vi "Input DMA Engine.vi"(8 "error in (no error)":errorcluster, 10 "Parameters":T1={"Waveform Ref"=refnum, "DMA Ref"=refnum, "Write to VS Engine.Refs"={"Refs"=[], "Values"=[]}, "Write to VS Engine.FIFO"=refnum, "Name"="", "DMA Settings"={"Number of Channels"=0, "Delacing Scheme"=enum."Interlaced", "Update Rate"=0, "dt"=1000.0}} {"DMA Settings"."dt" format="%#_p"; "DMA Settings"."Update Rate" items=["1 Hz"=1, "2 Hz"=2, "5 Hz"=5, "10 Hz"=10]; "Write to VS Engine.Refs"."Refs" format="%.0x"}, 11 "Parent":string) -> (0 "error out":errorcluster)   [LabVIEW 2015, in "FPGA Addon Engine.lvlib"]
uses:
  FPGA Addon Engine.lvlib
  Types/DMA Input References.ctl
  <vilib>/NI VeriStand/Custom Device Waveform API/Multiple Waveforms Write (DBL)/Multiple Waveforms Write (DBL).lvclass
  Types/DMA Input Ref.ctl
  <vilib>/NI Veristand/Custom Device API/Data Reference.ctl
  Shared/DMA Settings.ctl
  Shared/Delacing Scheme.ctl
  <vilib>/NI Veristand/Custom Device Waveform API/Multiple Waveforms Write (DBL)/NI VeriStand - Close Multiple Waveforms Write Session (DBL).vi
  <vilib>/FPGAPlugInAG/Dynamic/niLvFpga_Close_Dynamic.vi
  <vilib>/rvi/interface/nirviCloseFPGA/nirviCloseFPGA.xnode
  <vilib>/NI VeriStand/Custom Device Waveform API/NI_VS Custom Device Waveform API.lvlib
  Error Handling API/Error Handling API.lvlib
  <vilib>/NI Veristand/Custom Device Tools/Custom Device Utility Library/Custom Device Utility Library.lvlib
  Inline Async API/Inline Async API.lvlib
  <vilib>/NI VeriStand/Custom Device API/Custom Device API.lvlib
  Shared/FPGA Addon Shared.lvlib
panel:
  in  "stop":bool
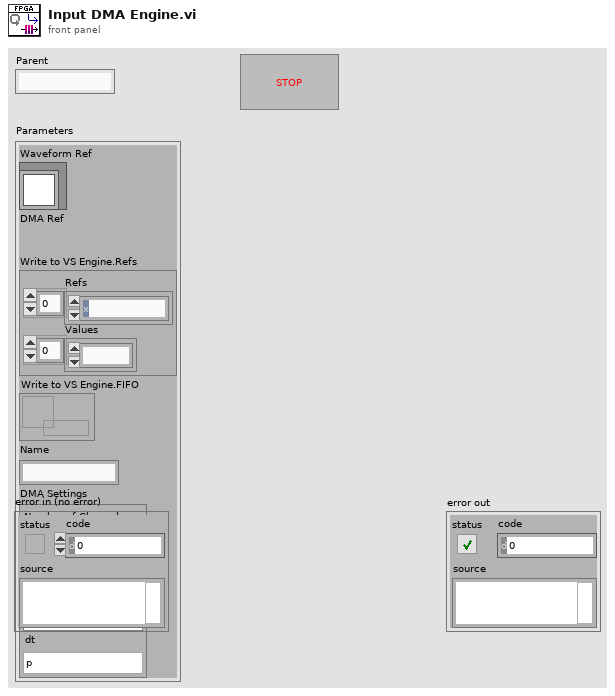
[diagram p1: front panel]
types:
  T1 = typedef "FPGA Addon Engine.lvlib/DMA Input References.ctl" = cluster{"Waveform Ref":refnum<class "Multiple Waveforms Write (DBL).lvclass">, "DMA Ref":T2, "Write to VS Engine.Refs":cluster{"Refs":T3[], "Values":dbl[]}, "Write to VS Engine.FIFO":refnum<k33>, "Name":string, "DMA Settings":T4}
  T2 = typedef "FPGA Addon Engine.lvlib/DMA Input Ref.ctl" = refnum<k20>
  T3 = typedef "Custom Device API.lvlib/Data Reference.ctl" = i32
  T4 = typedef "FPGA Addon Shared.lvlib/DMA Settings.ctl" = cluster{"Number of Channels":u8, "Delacing Scheme":T5, "Update Rate":u32, "dt":dbl}
  T5 = typedef "FPGA Addon Shared.lvlib/Delacing Scheme.ctl" = enum8{"Interlaced"}
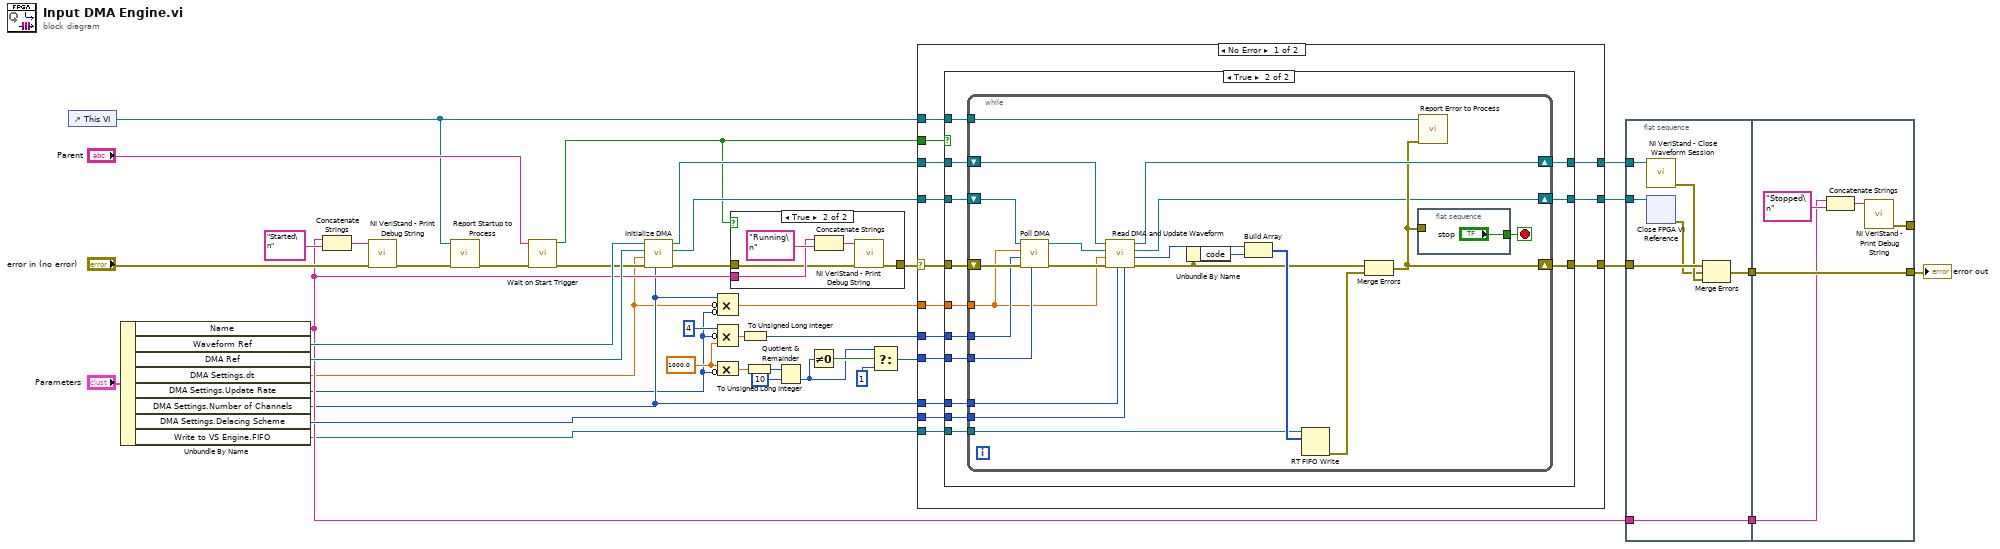
[diagram p0: block diagram]
diagram:
  w6 = 1000.0 ("y")
  n1 = control-ref of="This VI"() -> (w32:refnum<vi>)
  n2 = Unbundle By Name("Parameters") -> ("Name"=w10:string, "Waveform Ref"=w39:refnum<class "Multiple Waveforms Write (DBL).lvclass">, "DMA Ref"=w18:T2, "DMA Settings.dt"=w3:dbl, "DMA Settings.Update Rate"=w2:u32, "DMA Settings.Number of Channels"=w4:u8, "DMA Settings.Delacing Scheme"=w19:T5, "Write to VS Engine.FIFO"=w9:refnum<k33>)
  n3 = Concatenate Strings(w10, "Started\n" ("string")) -> (w29:string)
  n4 = call <vilib>:"NI VeriStand - Print Debug String.vi"("error in (no error)"="error in (no error)", "Message"=w29) -> ("error out"=w17:errorcluster)  [unwired: 9 in]
  n5 = call "Report Startup to Process.vi"("Error"=w17, "This VI"=w32) -> ("error out"=w31:errorcluster)  [unwired: 9 in]
  n6 = call "Wait on Start Trigger.vi"("error in (no error)"=w31, "Name"="Parent") -> ("error out"=w14:errorcluster, "notification"=w15:bool)  [unwired: 8 in]
  n7 = call "Initialize DMA.vi"("Number of Channels"=w4, "error in (no error)"=w14, "dt"=w3, "DMA Ref"=w18, "Multiple Waveforms Write (DBL) in"=w39) -> ("error out"=w13:errorcluster, "DMA Ref"=w37:T2, "Multiple Waveforms Write (DBL) out"=w38:refnum<class "Multiple Waveforms Write (DBL).lvclass">)  [unwired: 4 in]
  n8 = Compound Arithmetic op=MULTIPLY(w4, invert w3, invert w2) -> (w1:dbl)
  n9 = Compound Arithmetic op=MULTIPLY(u32 4 ("value"), invert w2, w6) -> (w7:dbl)
  n10 = Compound Arithmetic op=MULTIPLY(w6, invert w2) -> (w21:dbl)
  n11 = case shown="True" w15 {
    tunnel: w10 -> [_ w44]
    tunnel: w13 -> [w41 w43]
    tunnel: [w41 w42] -> w12
    frame False {
    }
    frame True {
      n12 = Concatenate Strings(w44, "Running\n" ("string")) -> (w46:string)
      n13 = call <vilib>:"NI VeriStand - Print Debug String.vi"("error in (no error)"=w43, "Message"=w46) -> ("error out"=w42:errorcluster)  [unwired: 9 in]
    }
  }
  n14 = To Unsigned Long Integer(number=w7) -> (unsigned 32bit integer=w5:u32)
  n15 = To Unsigned Long Integer(number=w21) -> (unsigned 32bit integer=w24:u32)
  n16 = Quotient & Remainder(x=w24, y=u32 10) -> (floor(x/y)=w20:u32)  [unwired: 1 out]
  n17 = Not Equal To 0?(x=w20) -> (x != 0?=w27:bool)
  n18 = Select(t=w20, s=w27, f=u32 1) -> (s? t:f=w8:u32)
  n19 = case shown="No Error" w12 {
    selector: w12 -> [w52 w101]
    tunnel: w38 -> [w60 w100]
    tunnel: w37 -> [w59 w99]
    tunnel: w1 -> [w58 _]
    tunnel: w4 -> [w57 _]
    tunnel: [w56 w100] -> w36
    tunnel: [w55 w101] -> w35
    tunnel: w5 -> [w54 _]
    tunnel: w32 -> [w53 _]
    tunnel: w15 -> [w51 _]
    tunnel: w8 -> [w50 _]
    tunnel: [w49 w99] -> w23
    tunnel: w19 -> [w48 _]
    tunnel: w9 -> [w47 _]
    frame No Error {
      n20 = case shown="True" w51 {
        tunnel: w60 -> [w63 w76]
        tunnel: w59 -> [w61 w75]
        tunnel: w58 -> [_ w74]
        tunnel: w57 -> [_ w73]
        tunnel: [w63 w72] -> w56
        tunnel: [w62 w71] -> w55
        tunnel: w54 -> [_ w70]
        tunnel: w53 -> [_ w69]
        tunnel: w52 -> [w62 w68]
        tunnel: w50 -> [_ w67]
        tunnel: [w61 w66] -> w49
        tunnel: w48 -> [_ w65]
        tunnel: w47 -> [_ w64]
        frame False {
        }
        frame True {
          n21 = while {
            shift-right: [w84] -> w71
            shift-left: w68 -> [w95]
            tunnel: w70 -> [w93]
            tunnel: w74 -> [w80]
            tunnel: w73 -> [w79]
            tunnel: w69 -> [w91]
            tunnel: w67 -> [w89]
            tunnel: w65 -> [w78]
            tunnel: w64 -> [w86]
            shift-right: [w82] -> w66
            shift-left: w75 -> [w94]
            shift-right: [w92] -> w72
            shift-left: w76 -> [w96]
            stop <- w97 stop-if-true
            n22 = call "Poll DMA.vi"("Wait (ms)"=w89, "error in (no error)"=w95, "Timeout (ms)"=w93, "Total Samples to Read"=w80, "DMA Ref"=w94) -> ("error out"=w90:errorcluster, "DMA Ref"=w81:T2)  [unwired: 5 in]
            n23 = call "Read DMA and Update Waveform.vi"("Delacing Scheme"=w78, "Number of Channels"=w79, "error in (no error)"=w90, "Total Samples"=w80, "DMA Ref"=w81, "Multiple Waveforms Write (DBL) in"=w96) -> ("error out"=w77:errorcluster, "Elements Remaining"=w83:u32, "FPGA VI Reference Out"=w82:T2, "Multiple Waveforms Write (DBL) out"=w92:refnum<class "Multiple Waveforms Write (DBL).lvclass">)  [unwired: 2 in]
            n24 = Unbundle By Name(w77) -> ("code"=w88:i32)
            n25 = Build Array(w83, w88) -> (w87:u32[])
            n26 = RT FIFO Write(0:w86, 1:w87) -> (11:w85:errorcluster)  [unwired: 3 in, 3 out]
            n27 = Merge Errors(w77, w85) -> (w84:errorcluster)
            n28 = flat-sequence {
              tunnel: ["stop"] -> w97
              tunnel: w84 -> [_]
              frame #0 {
              }
            }
            n29 = call "Report Error to Process.vi"("Error"=w84, "This VI"=w91) -> ()  [unwired: 10 in]
          }
        }
      }
    }
    frame Error {
    }
  }
  n30 = flat-sequence {
    tunnel: w36 -> [w108]
    tunnel: w35 -> [w107]
    tunnel: w23 -> [w104]
    tunnel: [w105] -> w16
    tunnel: [w102] -> w11
    tunnel: w10 -> [w102]
    tunnel: [w113] -> w22
    tunnel: w16 -> [w113]
    tunnel: w11 -> [w110]
    tunnel: [w109] -> _
    frame #0 {
      n31 = call-poly <vilib>:"NI VeriStand - Close Waveform Session.vi"("Multiple Waveforms Write Session (DBL)"=w108) -> ("error out"=w106:errorcluster)  [unwired: 10 in]
      n32 = xnode "Close FPGA VI Reference"("FPGA VI Reference In"=w104) -> ("error out"=w103:errorcluster)  [unwired: 1 in]
      n33 = Merge Errors(w107, w103, w106) -> (w105:errorcluster)
    }
    frame #1 {
      n34 = Concatenate Strings(w110, "Stopped\n" ("string")) -> (w111:string)
      n35 = call <vilib>:"NI VeriStand - Print Debug String.vi"("Message"=w111) -> ("error out"=w109:errorcluster)  [unwired: 10 in]
    }
  }
  "error out" <- w22
